vi "Calculadora.vi"() -> ()   [LabVIEW 2017]
uses:
  <vilib>/gmath/NI_Gmath.lvlib
panel:
  in  "Variable":i8
  out "ANS":string
  in  "Pantalla":string
  in  ")":bool
  in  "%":bool
  in  "Rad":bool
  in  "(":bool
  in  "e":bool
  in  "X^3":bool
  in  "1/x":bool
  in  "e^x":bool
  in  "X^2":bool
  in  "X^y":bool
  in  "Tanh":bool
  in  "Sqr":bool
  in  "X!":bool
  in  "Cosh":bool
  in  "Sinh":bool
  in  "Tan":bool
  in  "Ln":bool
  in  "Log":bool
  in  "Cos":bool
  in  "Sin":bool
  in  "Pi":bool
  in  "3":bool
  in  "6":bool
  in  "9":bool
  in  "Igual":bool
  in  "resta":bool
  in  "Div":bool
  in  "AC":bool
  in  "AnS":bool
  in  "suma":bool
  in  "multi":bool
  in  "del":bool
  in  ".":bool
  in  "2":bool
  in  "5":bool
  in  "8":bool
  in  "0":bool
  in  "1":bool
  in  "4":bool
  in  "7":bool
  # "CASIO"
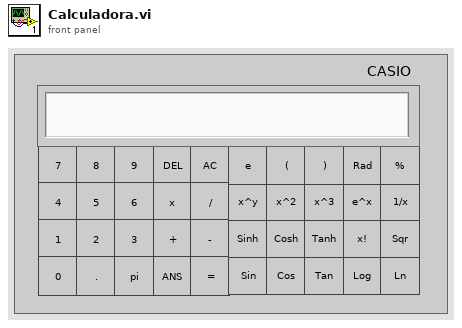
[diagram p1: front panel]
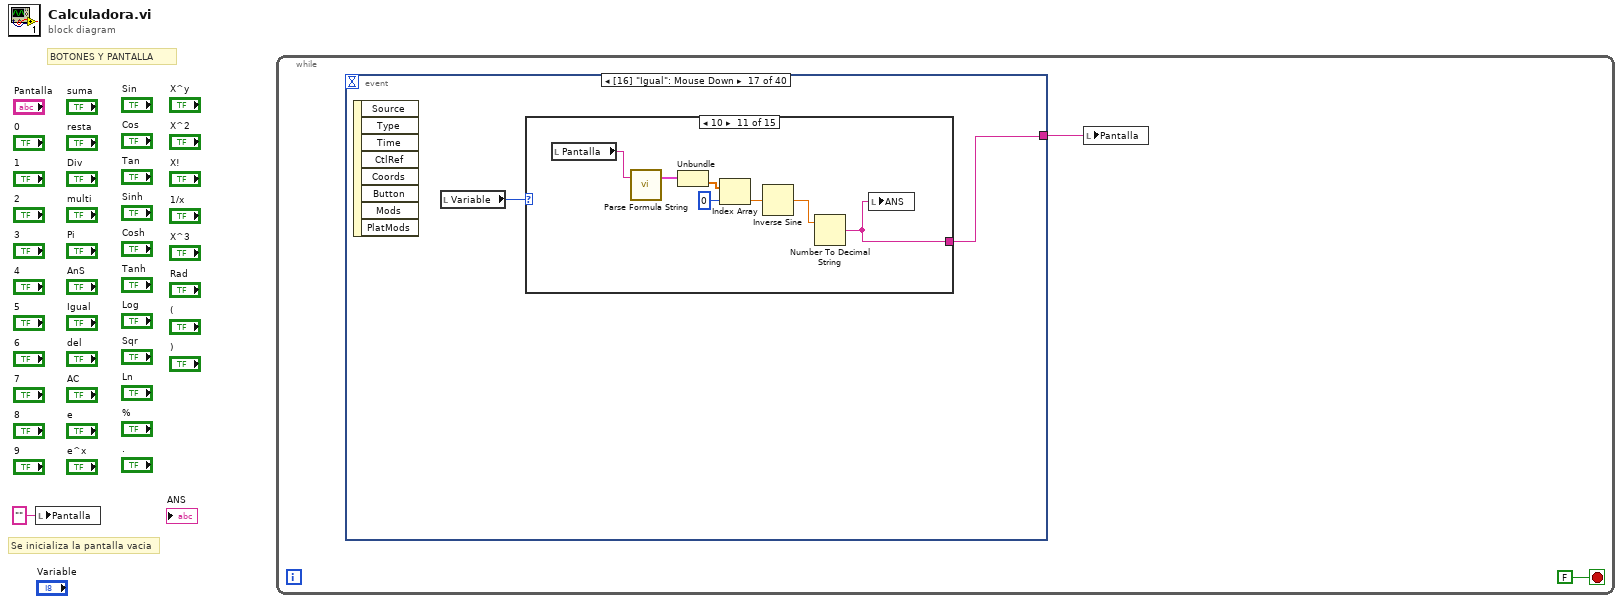
[diagram p0: block diagram]
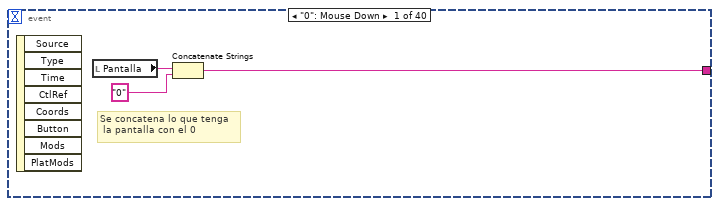
[diagram p2: hidden frame]
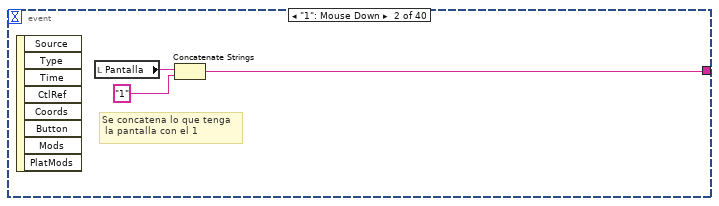
[diagram p3: hidden frame]
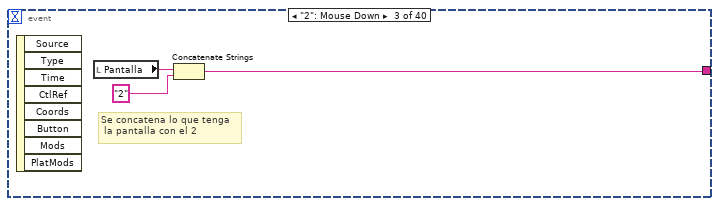
[diagram p4: hidden frame]
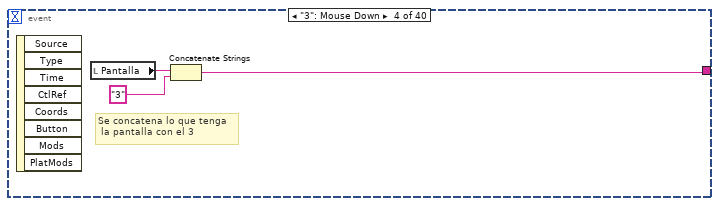
[diagram p5: hidden frame]
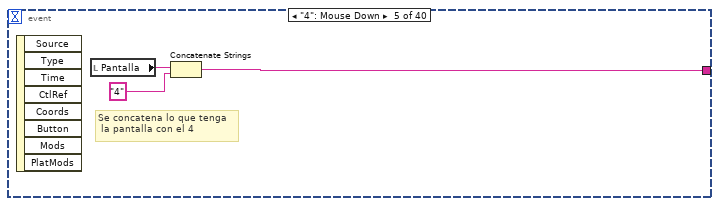
[diagram p6: hidden frame]
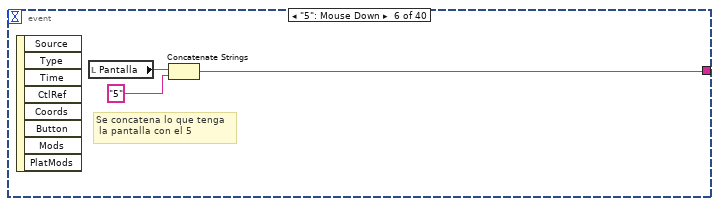
[diagram p7: hidden frame]
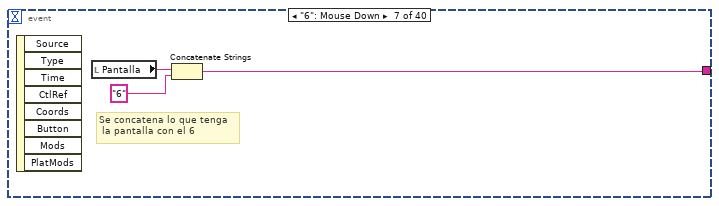
[diagram p8: hidden frame]
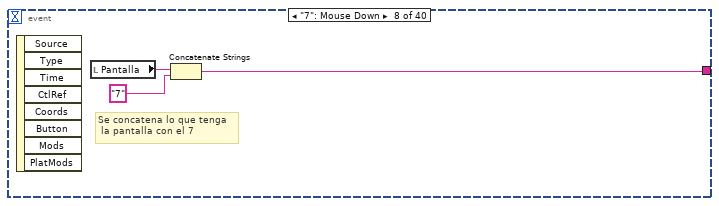
[diagram p9: hidden frame]
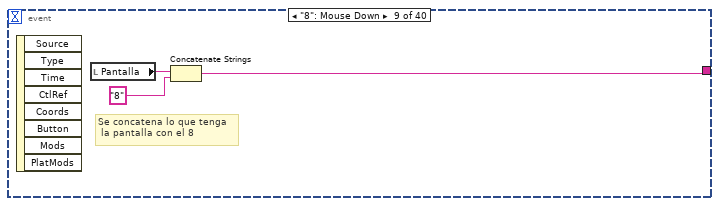
[diagram p10: hidden frame]
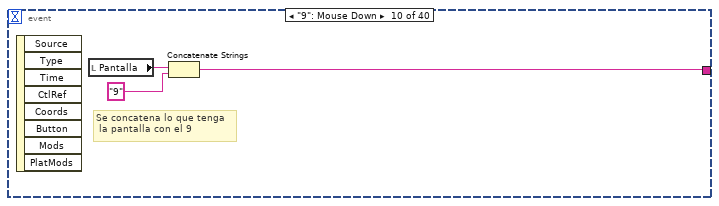
[diagram p11: hidden frame]
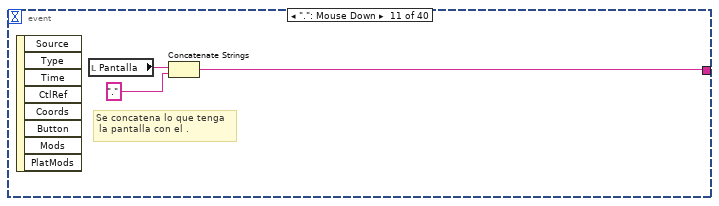
[diagram p12: hidden frame]
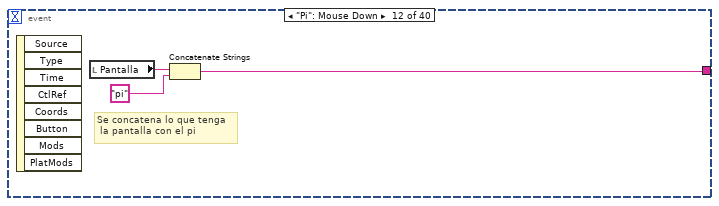
[diagram p13: hidden frame]
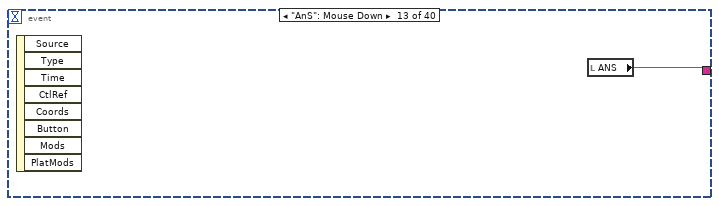
[diagram p14: hidden frame]
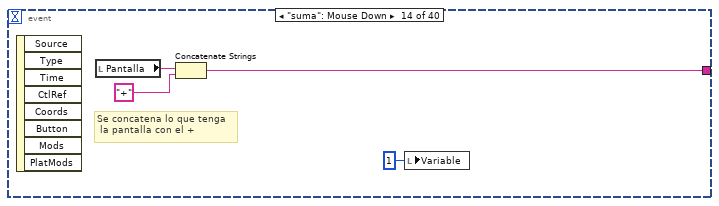
[diagram p15: hidden frame]
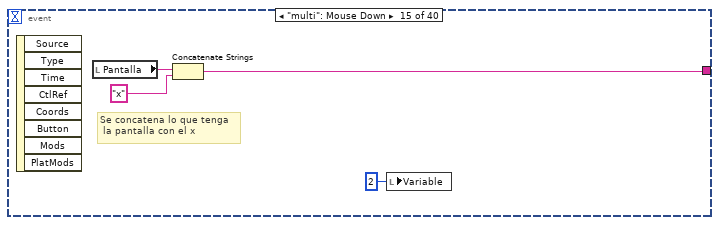
[diagram p16: hidden frame]
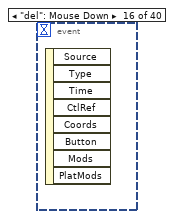
[diagram p17: hidden frame]
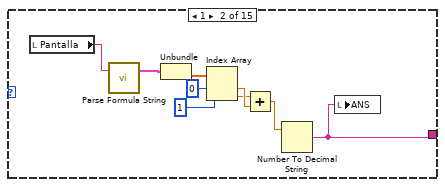
[diagram p19: hidden frame]
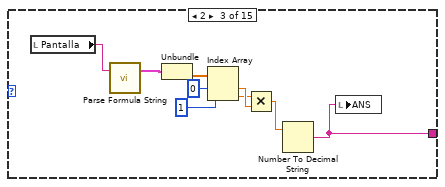
[diagram p20: hidden frame]
diagram:
  # "Se inicializa la pantalla vacia"
  # "BOTONES Y PANTALLA"
  n1 = local write "Pantalla"("" ("Pantalla")) -> ()
  n2 = while {
    stop <- FALSE stop-if-true
    n3 = event shown="[16] \"Igual\": Mouse Down" {
      selector: _ -> [_ _ _ _ _ _ _ _ _ _ _ _ _ _ _ _ _ _ _ _ _ _ _ _ _ _ _ _ _ _ _ _ _ _ _ _ _ _ _ _]
      dyn-events: _ -> [_ _ _ _ _ _ _ _ _ _ _ _ _ _ _ _ _ _ _ _ _ _ _ _ _ _ _ _ _ _ _ _ _ _ _ _ _ _ _ _]
      timeout: _ -> [_ _ _ _ _ _ _ _ _ _ _ _ _ _ _ _ _ _ _ _ _ _ _ _ _ _ _ _ _ _ _ _ _ _ _ _ _ _ _ _]
      tunnel: [w4 w7 w10 w13 w16 w19 w22 w25 w28 w31 w34 w37 w40 w42 w46 _ w49 w158 w162 _ w167 w171 w176 w181 w186 w191 w195 w200 w205 w209 _ w213 w217 w220 w223 w227 w230 _ w233 w236] -> w2
      event "0": Mouse Down {
        # "Se concatena lo que tenga\n la pantalla con el 0"
        n4 = event-data() -> ()  [unwired: 1 in, 8 out]
        n5 = local read "Pantalla"() -> (w6:string)
        n6 = Concatenate Strings(w6, "0") -> (w4:string)
      }
      event "1": Mouse Down {
        # "Se concatena lo que tenga\n la pantalla con el 1"
        n7 = event-data() -> ()  [unwired: 1 in, 8 out]
        n8 = local read "Pantalla"() -> (w9:string)
        n9 = Concatenate Strings(w9, "1") -> (w7:string)
      }
      event "2": Mouse Down {
        # "Se concatena lo que tenga\n la pantalla con el 2"
        n10 = event-data() -> ()  [unwired: 1 in, 8 out]
        n11 = local read "Pantalla"() -> (w12:string)
        n12 = Concatenate Strings(w12, "2") -> (w10:string)
      }
      event "3": Mouse Down {
        # "Se concatena lo que tenga\n la pantalla con el 3"
        n13 = event-data() -> ()  [unwired: 1 in, 8 out]
        n14 = local read "Pantalla"() -> (w15:string)
        n15 = Concatenate Strings(w15, "3") -> (w13:string)
      }
      event "4": Mouse Down {
        # "Se concatena lo que tenga\n la pantalla con el 4"
        n16 = event-data() -> ()  [unwired: 1 in, 8 out]
        n17 = local read "Pantalla"() -> (w18:string)
        n18 = Concatenate Strings(w18, "4") -> (w16:string)
      }
      event "5": Mouse Down {
        # "Se concatena lo que tenga\n la pantalla con el 5"
        n19 = event-data() -> ()  [unwired: 1 in, 8 out]
        n20 = local read "Pantalla"() -> (w21:string)
        n21 = Concatenate Strings(w21, "5") -> (w19:string)
      }
      event "6": Mouse Down {
        # "Se concatena lo que tenga\n la pantalla con el 6"
        n22 = event-data() -> ()  [unwired: 1 in, 8 out]
        n23 = local read "Pantalla"() -> (w24:string)
        n24 = Concatenate Strings(w24, "6") -> (w22:string)
      }
      event "7": Mouse Down {
        # "Se concatena lo que tenga\n la pantalla con el 7"
        n25 = event-data() -> ()  [unwired: 1 in, 8 out]
        n26 = local read "Pantalla"() -> (w27:string)
        n27 = Concatenate Strings(w27, "7") -> (w25:string)
      }
      event "8": Mouse Down {
        # "Se concatena lo que tenga\n la pantalla con el 8"
        n28 = event-data() -> ()  [unwired: 1 in, 8 out]
        n29 = local read "Pantalla"() -> (w30:string)
        n30 = Concatenate Strings(w30, "8") -> (w28:string)
      }
      event "9": Mouse Down {
        # "Se concatena lo que tenga\n la pantalla con el 9"
        n31 = event-data() -> ()  [unwired: 1 in, 8 out]
        n32 = local read "Pantalla"() -> (w33:string)
        n33 = Concatenate Strings(w33, "9") -> (w31:string)
      }
      event ".": Mouse Down {
        # "Se concatena lo que tenga\n la pantalla con el ."
        n34 = event-data() -> ()  [unwired: 1 in, 8 out]
        n35 = local read "Pantalla"() -> (w36:string)
        n36 = Concatenate Strings(w36, ".") -> (w34:string)
      }
      event "Pi": Mouse Down {
        # "Se concatena lo que tenga\n la pantalla con el pi"
        n37 = event-data() -> ()  [unwired: 1 in, 8 out]
        n38 = local read "Pantalla"() -> (w39:string)
        n39 = Concatenate Strings(w39, "pi") -> (w37:string)
      }
      event "AnS": Mouse Down {
        n40 = event-data() -> ()  [unwired: 1 in, 8 out]
        n41 = local read "ANS"() -> (w40:string)
      }
      event "suma": Mouse Down {
        # "Se concatena lo que tenga\n la pantalla con el +"
        n42 = event-data() -> ()  [unwired: 1 in, 8 out]
        n43 = local read "Pantalla"() -> (w44:string)
        n44 = Concatenate Strings(w44, "+") -> (w42:string)
        n45 = local write "Variable"(i8 1 ("Variable")) -> ()
      }
      event "multi": Mouse Down {
        # "Se concatena lo que tenga\n la pantalla con el x"
        n46 = event-data() -> ()  [unwired: 1 in, 8 out]
        n47 = local read "Pantalla"() -> (w48:string)
        n48 = Concatenate Strings(w48, "x") -> (w46:string)
        n49 = local write "Variable"(i8 2 ("Variable")) -> ()
      }
      event "del": Mouse Down {
        n50 = event-data() -> ()  [unwired: 1 in, 8 out]
      }
      event "Igual": Mouse Down {
        n51 = event-data() -> ()  [unwired: 1 in, 8 out]
        n52 = local read "Variable"() -> (w50:i8)
        n53 = case shown="10" w50 {
          tunnel: [_ w52 w60 w69 w78 w87 w94 w101 w108 w115 w122 w129 w136 w147 w150] -> w49
          frame 0, Default {
          }
          frame 1 {
            n54 = local read "Pantalla"() -> (w51:string)
            n55 = call <vilib>:"Parse Formula String.vi"("formula"=w51) -> ("Parsed Formula"=w53:cluster{"Table":i32[][], "Y Values":dbl[]})  [unwired: 1 in, 1 out]
            n56 = Unbundle(w53) -> ("Y Values"=w54:dbl[])  [unwired: 1 out]
            n57 = Index Array(array=w54, index #1=0 ("index"), index #2=1 ("index")) -> (element #1=w58:dbl, element #2=w57:dbl)
            n58 = Add(x=w57, y=w58) -> (x+y=w59:dbl)
            n59 = Number To Decimal String(number=w59) -> (decimal integer string=w52:string)  [unwired: 1 in]
            n60 = local write "ANS"(w52) -> ()
          }
          frame 2 {
            n61 = local read "Pantalla"() -> (w61:string)
            n62 = call <vilib>:"Parse Formula String.vi"("formula"=w61) -> ("Parsed Formula"=w62:cluster{"Table":i32[][], "Y Values":dbl[]})  [unwired: 1 in, 1 out]
            n63 = Unbundle(w62) -> ("Y Values"=w63:dbl[])  [unwired: 1 out]
            n64 = Index Array(array=w63, index #1=0 ("index"), index #2=1 ("index")) -> (element #1=w67:dbl, element #2=w66:dbl)
            n65 = Multiply(x=w66, y=w67) -> (x*y=w68:dbl)
            n66 = Number To Decimal String(number=w68) -> (decimal integer string=w60:string)  [unwired: 1 in]
            n67 = local write "ANS"(w60) -> ()
          }
          frame 3 {
            n68 = local read "Pantalla"() -> (w70:string)
            n69 = call <vilib>:"Parse Formula String.vi"("formula"=w70) -> ("Parsed Formula"=w71:cluster{"Table":i32[][], "Y Values":dbl[]})  [unwired: 1 in, 1 out]
            n70 = Unbundle(w71) -> ("Y Values"=w72:dbl[])  [unwired: 1 out]
            n71 = Index Array(array=w72, index #1=0 ("index"), index #2=1 ("index")) -> (element #1=w76:dbl, element #2=w75:dbl)
            n72 = Subtract(x=w75, y=w76) -> (x-y=w77:dbl)
            n73 = Number To Decimal String(number=w77) -> (decimal integer string=w69:string)  [unwired: 1 in]
            n74 = local write "ANS"(w69) -> ()
          }
          frame 4 {
            n75 = local read "Pantalla"() -> (w79:string)
            n76 = call <vilib>:"Parse Formula String.vi"("formula"=w79) -> ("Parsed Formula"=w80:cluster{"Table":i32[][], "Y Values":dbl[]})  [unwired: 1 in, 1 out]
            n77 = Unbundle(w80) -> ("Y Values"=w81:dbl[])  [unwired: 1 out]
            n78 = Index Array(array=w81, index #1=0 ("index"), index #2=1 ("index")) -> (element #1=w85:dbl, element #2=w84:dbl)
            n79 = Divide(x=w84, y=w85) -> (x/y=w86:dbl)
            n80 = Number To Decimal String(number=w86) -> (decimal integer string=w78:string)  [unwired: 1 in]
            n81 = local write "ANS"(w78) -> ()
          }
          frame 5 {
            n82 = local read "Pantalla"() -> (w93:string)
            n83 = call <vilib>:"Parse Formula String.vi"("formula"=w93) -> ("Parsed Formula"=w92:cluster{"Table":i32[][], "Y Values":dbl[]})  [unwired: 1 in, 1 out]
            n84 = Unbundle(w92) -> ("Y Values"=w91:dbl[])  [unwired: 1 out]
            n85 = Index Array(array=w91, index=0) -> (element=w89:dbl)
            n86 = Sine(x=w89) -> (sin(x)=w88:dbl)
            n87 = Number To Decimal String(number=w88) -> (decimal integer string=w87:string)  [unwired: 1 in]
            n88 = local write "ANS"(w87) -> ()
          }
          frame 6 {
            n89 = local read "Pantalla"() -> (w100:string)
            n90 = call <vilib>:"Parse Formula String.vi"("formula"=w100) -> ("Parsed Formula"=w99:cluster{"Table":i32[][], "Y Values":dbl[]})  [unwired: 1 in, 1 out]
            n91 = Unbundle(w99) -> ("Y Values"=w98:dbl[])  [unwired: 1 out]
            n92 = Index Array(array=w98, index=0) -> (element=w96:dbl)
            n93 = Cosine(x=w96) -> (cos(x)=w95:dbl)
            n94 = Number To Decimal String(number=w95) -> (decimal integer string=w94:string)  [unwired: 1 in]
            n95 = local write "ANS"(w94) -> ()
          }
          frame 7 {
            n96 = local read "Pantalla"() -> (w107:string)
            n97 = call <vilib>:"Parse Formula String.vi"("formula"=w107) -> ("Parsed Formula"=w106:cluster{"Table":i32[][], "Y Values":dbl[]})  [unwired: 1 in, 1 out]
            n98 = Unbundle(w106) -> ("Y Values"=w105:dbl[])  [unwired: 1 out]
            n99 = Index Array(array=w105, index=0) -> (element=w103:dbl)
            n100 = Tangent(1:w103) -> (0:w102:dbl)
            n101 = Number To Decimal String(number=w102) -> (decimal integer string=w101:string)  [unwired: 1 in]
            n102 = local write "ANS"(w101) -> ()
          }
          frame 8 {
            n103 = local read "Pantalla"() -> (w114:string)
            n104 = call <vilib>:"Parse Formula String.vi"("formula"=w114) -> ("Parsed Formula"=w113:cluster{"Table":i32[][], "Y Values":dbl[]})  [unwired: 1 in, 1 out]
            n105 = Unbundle(w113) -> ("Y Values"=w112:dbl[])  [unwired: 1 out]
            n106 = Index Array(array=w112, index=0) -> (element=w110:dbl)
            n107 = Logarithm Base 10(1:w110) -> (0:w109:dbl)
            n108 = Number To Decimal String(number=w109) -> (decimal integer string=w108:string)  [unwired: 1 in]
            n109 = local write "ANS"(w108) -> ()
          }
          frame 9 {
            n110 = local read "Pantalla"() -> (w121:string)
            n111 = call <vilib>:"Parse Formula String.vi"("formula"=w121) -> ("Parsed Formula"=w120:cluster{"Table":i32[][], "Y Values":dbl[]})  [unwired: 1 in, 1 out]
            n112 = Unbundle(w120) -> ("Y Values"=w119:dbl[])  [unwired: 1 out]
            n113 = Index Array(array=w119, index=0) -> (element=w117:dbl)
            n114 = Natural Logarithm(1:w117) -> (0:w116:dbl)
            n115 = Number To Decimal String(number=w116) -> (decimal integer string=w115:string)  [unwired: 1 in]
            n116 = local write "ANS"(w115) -> ()
          }
          frame 10 {
            n117 = local read "Pantalla"() -> (w128:string)
            n118 = call <vilib>:"Parse Formula String.vi"("formula"=w128) -> ("Parsed Formula"=w127:cluster{"Table":i32[][], "Y Values":dbl[]})  [unwired: 1 in, 1 out]
            n119 = Unbundle(w127) -> ("Y Values"=w126:dbl[])  [unwired: 1 out]
            n120 = Index Array(array=w126, index=0) -> (element=w124:dbl)
            n121 = Inverse Sine(1:w124) -> (0:w123:dbl)
            n122 = Number To Decimal String(number=w123) -> (decimal integer string=w122:string)  [unwired: 1 in]
            n123 = local write "ANS"(w122) -> ()
          }
          frame 11 {
            n124 = local read "Pantalla"() -> (w135:string)
            n125 = call <vilib>:"Parse Formula String.vi"("formula"=w135) -> ("Parsed Formula"=w134:cluster{"Table":i32[][], "Y Values":dbl[]})  [unwired: 1 in, 1 out]
            n126 = Unbundle(w134) -> ("Y Values"=w133:dbl[])  [unwired: 1 out]
            n127 = Index Array(array=w133, index=0) -> (element=w131:dbl)
            n128 = Inverse Cosine(1:w131) -> (0:w130:dbl)
            n129 = Number To Decimal String(number=w130) -> (decimal integer string=w129:string)  [unwired: 1 in]
            n130 = local write "ANS"(w129) -> ()
          }
          frame 12 {
            n131 = local read "Pantalla"() -> (w142:string)
            n132 = call <vilib>:"Parse Formula String.vi"("formula"=w142) -> ("Parsed Formula"=w141:cluster{"Table":i32[][], "Y Values":dbl[]})  [unwired: 1 in, 1 out]
            n133 = Unbundle(w141) -> ("Y Values"=w140:dbl[])  [unwired: 1 out]
            n134 = Index Array(array=w140, index=0) -> (element=w138:dbl)
            n135 = Inverse Tangent(1:w138) -> (0:w137:dbl)
            n136 = Number To Decimal String(number=w137) -> (decimal integer string=w136:string)  [unwired: 1 in]
            n137 = local write "ANS"(w136) -> ()
          }
          frame 13 {
            n138 = local read "Pantalla"() -> (w149:string)
            n139 = call <vilib>:"Parse Formula String.vi"("formula"=w149) -> ("Parsed Formula"=w148:cluster{"Table":i32[][], "Y Values":dbl[]})  [unwired: 1 in, 1 out]
            n140 = Unbundle(w148) -> ("Y Values"=w146:dbl[])  [unwired: 1 out]
            n141 = Index Array(array=w146, index=0) -> (element=w143:dbl)
            n142 = Square Root(x=w143) -> (sqrt(x)=w144:dbl)
            n143 = Number To Decimal String(number=w144) -> (decimal integer string=w147:string)  [unwired: 1 in]
            n144 = local write "ANS"(w147) -> ()
          }
          frame 14 {
            n145 = local read "Pantalla"() -> (w156:string)
            n146 = call <vilib>:"Parse Formula String.vi"("formula"=w156) -> ("Parsed Formula"=w155:cluster{"Table":i32[][], "Y Values":dbl[]})  [unwired: 1 in, 1 out]
            n147 = Unbundle(w155) -> ("Y Values"=w154:dbl[])  [unwired: 1 out]
            n148 = Index Array(array=w154, index=0) -> (element=w152:dbl)
            n149 = Square Root(x=w152) -> (sqrt(x)=w153:dbl)
            n150 = Number To Decimal String(number=w153) -> (decimal integer string=w150:string)  [unwired: 1 in]
            n151 = local write "ANS"(w150) -> ()
          }
        }
      }
      event "resta": Mouse Down {
        # "Se concatena lo que tenga\n la pantalla con el -"
        n152 = event-data() -> ()  [unwired: 1 in, 8 out]
        n153 = local read "Pantalla"() -> (w160:string)
        n154 = Concatenate Strings(w160, "-") -> (w158:string)
        n155 = local write "Variable"(i8 3 ("Variable")) -> ()
      }
      event "Div": Mouse Down {
        # "Se concatena lo que tenga\n la pantalla con el /"
        n156 = event-data() -> ()  [unwired: 1 in, 8 out]
        n157 = local read "Pantalla"() -> (w164:string)
        n158 = Concatenate Strings(w164, "/") -> (w162:string)
        n159 = local write "Variable"(i8 4 ("Variable")) -> ()
      }
      event "AC": Mouse Down {
        n160 = event-data() -> ()  [unwired: 1 in, 8 out]
      }
      event "Sin": Mouse Down {
        # "Se concatena lo que tenga\n la pantalla con el sin"
        n161 = event-data() -> ()  [unwired: 1 in, 8 out]
        n162 = local read "Pantalla"() -> (w169:string)
        n163 = Concatenate Strings(w169, "sin", "(") -> (w167:string)
        n164 = local write "Variable"(i8 5 ("Variable")) -> ()
      }
      event "Cos": Mouse Down {
        # "Se concatena lo que tenga\n la pantalla con el cos"
        n165 = event-data() -> ()  [unwired: 1 in, 8 out]
        n166 = local read "Pantalla"() -> (w174:string)
        n167 = Concatenate Strings(w174, "cos", "(") -> (w171:string)
        n168 = local write "Variable"(i8 6 ("Variable")) -> ()
      }
      event "Log": Mouse Down {
        # "Se concatena lo que tenga\n la pantalla con el log"
        n169 = event-data() -> ()  [unwired: 1 in, 8 out]
        n170 = local read "Pantalla"() -> (w179:string)
        n171 = Concatenate Strings(w179, "log", "(") -> (w176:string)
        n172 = local write "Variable"(i8 8 ("Variable")) -> ()
      }
      event "Ln": Mouse Down {
        # "Se concatena lo que tenga\n la pantalla con el ln"
        n173 = event-data() -> ()  [unwired: 1 in, 8 out]
        n174 = local read "Pantalla"() -> (w184:string)
        n175 = Concatenate Strings(w184, "ln", "(") -> (w181:string)
        n176 = local write "Variable"(i8 9 ("Variable")) -> ()
      }
      event "Tan": Mouse Down {
        # "Se concatena lo que tenga\n la pantalla con el tan"
        n177 = event-data() -> ()  [unwired: 1 in, 8 out]
        n178 = local read "Pantalla"() -> (w189:string)
        n179 = Concatenate Strings(w189, "tan", "(") -> (w186:string)
        n180 = local write "Variable"(i8 7 ("Variable")) -> ()
      }
      event "Sinh": Mouse Down {
        # "Se concatena lo que tenga\n la pantalla con el sinh"
        n181 = event-data() -> ()  [unwired: 1 in, 8 out]
        n182 = local read "Pantalla"() -> (w193:string)
        n183 = Concatenate Strings(w193, "arcsin") -> (w191:string)
        n184 = local write "Variable"(i8 10 ("Variable")) -> ()
      }
      event "Cosh": Mouse Down {
        # "Se concatena lo que tenga\n la pantalla con el cos"
        n185 = event-data() -> ()  [unwired: 1 in, 8 out]
        n186 = local read "Pantalla"() -> (w198:string)
        n187 = Concatenate Strings(w198, "cosh", "(") -> (w195:string)
        n188 = local write "Variable"(i8 11 ("Variable")) -> ()
      }
      event "X!": Mouse Down {
        # "Se concatena lo que tenga\n la pantalla con el x!"
        n189 = event-data() -> ()  [unwired: 1 in, 8 out]
        n190 = local read "Pantalla"() -> (w202:string)
        n191 = Concatenate Strings(w202, "fp") -> (w200:string)
        n192 = local write "Variable"(i8 14 ("Variable")) -> ()
      }
      event "Sqr": Mouse Down {
        # "Se concatena lo que tenga\n la pantalla con el logx"
        n193 = event-data() -> ()  [unwired: 1 in, 8 out]
        n194 = local read "Pantalla"() -> (w207:string)
        n195 = Concatenate Strings(w207, "square", "(" ("string")) -> (w205:string)
        n196 = local write "Variable"(i8 13 ("Variable")) -> ()
      }
      event "Tanh": Mouse Down {
        # "Se concatena lo que tenga\n la pantalla con el tanh"
        n197 = event-data() -> ()  [unwired: 1 in, 8 out]
        n198 = local read "Pantalla"() -> (w212:string)
        n199 = Concatenate Strings(w212, "tanh", "(") -> (w209:string)
        n200 = local write "Variable"(i8 12 ("Variable")) -> ()
      }
      event "X^y": Mouse Down {
        n201 = event-data() -> ()  [unwired: 1 in, 8 out]
      }
      event "X^2": Mouse Down {
        # "Se concatena lo que tenga\n la pantalla con el x^2"
        n202 = event-data() -> ()  [unwired: 1 in, 8 out]
        n203 = local read "Pantalla"() -> (w216:string)
        n204 = Concatenate Strings(w216, "^", "2") -> (w213:string)
      }
      event "e^x": Mouse Down {
        # "Se concatena lo que tenga\n la pantalla con el e^x"
        n205 = event-data() -> ()  [unwired: 1 in, 8 out]
        n206 = local read "Pantalla"() -> (w219:string)
        n207 = Concatenate Strings(w219, "e^") -> (w217:string)
      }
      event "1/x": Mouse Down {
        # "Se concatena lo que tenga\n la pantalla con el 1/x"
        n208 = event-data() -> ()  [unwired: 1 in, 8 out]
        n209 = local read "Pantalla"() -> (w222:string)
        n210 = Concatenate Strings(w222, "1/") -> (w220:string)
      }
      event "X^3": Mouse Down {
        # "Se concatena lo que tenga\n la pantalla con el x^3"
        n211 = event-data() -> ()  [unwired: 1 in, 8 out]
        n212 = local read "Pantalla"() -> (w226:string)
        n213 = Concatenate Strings(w226, "^", "3") -> (w223:string)
      }
      event "e": Mouse Down {
        # "Se concatena lo que tenga\n la pantalla con el e"
        n214 = event-data() -> ()  [unwired: 1 in, 8 out]
        n215 = local read "Pantalla"() -> (w229:string)
        n216 = Concatenate Strings(w229, "e") -> (w227:string)
      }
      event "(": Mouse Down {
        # "Se concatena lo que tenga\n la pantalla con el ("
        n217 = event-data() -> ()  [unwired: 1 in, 8 out]
        n218 = local read "Pantalla"() -> (w232:string)
        n219 = Concatenate Strings(w232, "(") -> (w230:string)
      }
      event "Rad": Mouse Down {
        n220 = event-data() -> ()  [unwired: 1 in, 8 out]
      }
      event "%": Mouse Down {
        # "Se concatena lo que tenga\n la pantalla con el %"
        n221 = event-data() -> ()  [unwired: 1 in, 8 out]
        n222 = local read "Pantalla"() -> (w235:string)
        n223 = Concatenate Strings(w235, "%") -> (w233:string)
      }
      event ")": Mouse Down {
        # "Se concatena lo que tenga\n la pantalla con el )"
        n224 = event-data() -> ()  [unwired: 1 in, 8 out]
        n225 = local read "Pantalla"() -> (w238:string)
        n226 = Concatenate Strings(w238, ")") -> (w236:string)
      }
    }
    n227 = local write "Pantalla"(w2) -> ()
  }
